vi "保存数据记录文件.vi"() -> ()   [LabVIEW 2010]
uses:
  <vilib>/Analysis/NI_AALBase.lvlib
panel:
  out "数据记录":cluster{"采样时间":string, "采样率":dbl, "采样数据":dbl[]} {"采样数据" format="%.2f"; "采样率" format="%.2f"}
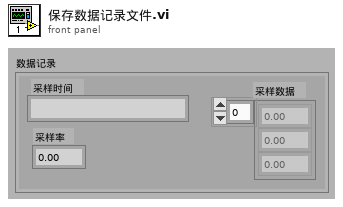
[diagram p1: front panel]
types:
  T1 = enum16{"open", "replace", "create", "open or create", "replace or create", "replace or create with confirmation"}
  T2 = cluster{"date/time string":string, "采样率":dbl, "sine wave":dbl[]}
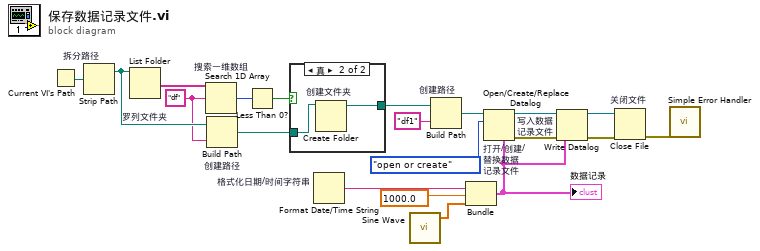
[diagram p0: block diagram]
diagram:
  w6 = "df"
  n1 = Current VI's Path() -> (path=w12:path)
  n2 = Strip Path "拆分路径"(path=w12) -> (stripped path=w7:path)  [unwired: 1 out]
  n3 = List Folder "罗列文件夹"(path=w7) -> (folder names=w11:string[])  [unwired: 3 in, 3 out]
  n4 = Search 1D Array "搜索一维数组"(1D array=w11, element=w6) -> (index of element=w10:i32)  [unwired: 1 in]
  n5 = Build Path "创建路径"(base path=w7, name or relative path=w6) -> (appended path=w5:path)
  n6 = Less Than 0?(x=w10) -> (x < 0?=w8:bool)
  n7 = case shown="真" w8 {
    tunnel: w5 -> [w21 w23]
    tunnel: [w21 w22] -> w4
    frame False {
    }
    frame True {
      n8 = Create Folder "创建文件夹"(path (use dialog)=w23) -> (created path=w22:path)  [unwired: 2 in, 2 out]
    }
  }
  n9 = Format Date/Time String "格式化日期/时间字符串"() -> (date/time string=w17:string)  [unwired: 3 in]
  n10 = call <vilib>:"Sine Wave.vi"() -> ("sine wave"=w16:dbl[])  [unwired: 5 in, 2 out]
  n11 = Build Path "创建路径"(base path=w4, name or relative path="df1") -> (appended path=w3:path)
  n12 = Bundle("date/time string"=w17, "采样率"=1000.0, "sine wave"=w16) -> (w13:T2)  [unwired: 1 in]
  "数据记录" <- w13
  n13 = Open/Create/Replace Datalog "打开/创建/\n替换数据\n记录文件"(5:w13, 10:T1."open or create" ("操作(0:open)"), 11:w3) -> (0:w20:errorcluster, 3:w14:refnum<k1>)  [unwired: 3 in, 1 out]
  n14 = Write Datalog "写入数据\n记录文件"(4:w20, 6:w13, 7:w14) -> (0:w18:errorcluster, 3:w19:refnum<k1>)
  n15 = Close File "关闭文件"(refnum=w19, error in=w18) -> (error out=w15:errorcluster)  [unwired: 1 out]
  n16 = call <vilib>:"Simple Error Handler.vi"("error in (no error)"=w15) -> ()  [unwired: 4 in, 5 out]
